vi "workbook get worksheet by name lv.vi"(8 "error in (no error)":errorcluster, 10 "name":string, 11 "workbook":u32) -> (0 "error out":errorcluster, 3 "function return":u32)   [LabVIEW 8.6]
doc: "lxw_worksheet workbook_get_worksheet_by_name_lv(lxw_workbook workbook, const char *name);"
uses:
  pending_lvxlsxwriter/xlsxwriter.dll
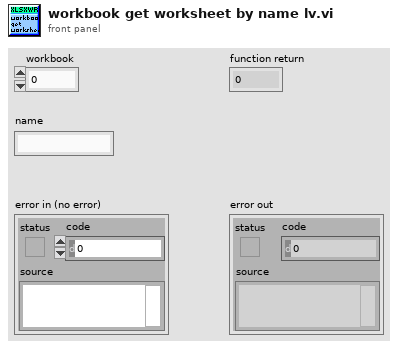
[diagram p1: front panel]
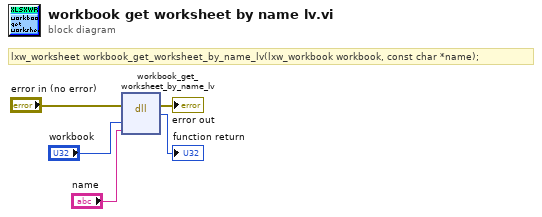
[diagram p0: block diagram]
diagram:
  # "lxw_worksheet workbook_get_worksheet_by_name_lv(lxw_workbook workbook, const char *name);"
  n1 = dll-call lib="C:/Users/WDAGUtilityAccount/Desktop/pending_lvxlsxwriter/xlsxwriter.*" fn="workbook_get_worksheet_by_name_lv"(error in="error in (no error)", "workbook"="workbook", "name"="name") -> (error out=→"error out":errorcluster, →"function return":u32)  [unwired: 4 in, 1 out]
